vi "Read Ordered deps.vi"(9 "length (-1)":i32=-1, 10 "index":i32, 11 "BuildManager in":refnum<class "BuildManager.lvclass">) -> (2 "Ordered deps":refnum<class "ProjectItem.lvclass">[](array[class]), 3 "BuildManager out":refnum<class "BuildManager.lvclass">)   [LabVIEW 2020, in "SolutionBuilder.lvlib" / "BuildManager.lvclass"]
uses:
  BuildManager.lvclass
  ProjectItem/ProjectItem.lvclass
  BuildManager.lvclass/BuildManager.ctl
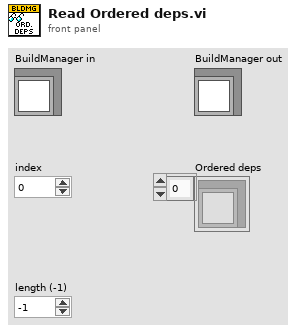
[diagram p1: front panel]
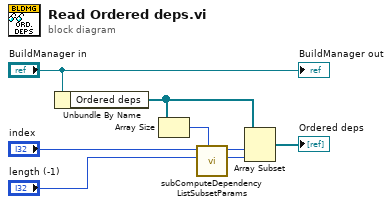
[diagram p0: block diagram]
diagram:
  n1 = Unbundle By Name("BuildManager in") -> ("Ordered deps"=w6:refnum<class "ProjectItem.lvclass">[])
  n2 = Array Size(array=w6) -> (size(s)=w1:i32)
  n3 = call "subComputeDependencyListSubsetParams.vi"("size"=w1, "length (-1)"="length (-1)", "index"="index") -> ("length out"=w5:i32, "index out"=w4:i32)  [unwired: 7 in]
  n4 = Array Subset(array=w6, index=w4, length=w5) -> (→"Ordered deps":refnum<class "ProjectItem.lvclass">[])
  "BuildManager out" <- "BuildManager in"
